vi "GetMUXRelayInfo.vi"(8 "error in (no error)":errorcluster, 10 "gRPCid":T2, 11 "ctet_mux in":T1) -> (0 "error out":errorcluster, 3 "ctet_mux out":T1)   [LabVIEW 2019, in "ctet_mux_User Library.lvlib"]
uses:
  ctet_mux_User Library.lvlib
  Servers/ctet_mux/gRPC lvSupport/Server API/typeDefs/grpcId.ctl
  Types/ctet_mux.ctl
  Servers/ctet_mux/ctet_mux Class/RPC Messages/measurementservice_MUXGetRelayInfoResponse/measurementservice_MUXGetRelayInfoResponse_Data.ctl
  Servers/ctet_mux/ctet_mux Class/RPC Messages/measurementservice_RelayInfoCluster/measurementservice_RelayInfoCluster_Data.ctl
  Servers/ctet_mux/ctet_mux Class/RPC Messages/measurementservice_ErrorOut/measurementservice_ErrorOut_Data.ctl
  Servers/ctet_mux/ctet_mux Class/ctet_mux.lvclass
  Servers/ctet_mux/gRPC lvSupport/gprc-lvsupport.lvlib
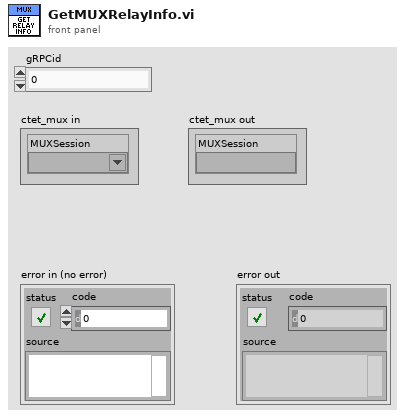
[diagram p1: front panel]
types:
  T1 = typedef "ctet_mux_User Library.lvlib/ctet_mux.ctl" = cluster{"MUXSession":refnum<k15>}
  T2 = typedef "ctet_mux.lvlib/gprc-lvsupport.lvlib/grpcId.ctl" = u64
  T3 = typedef "ctet_mux.lvlib/ctet_mux.lvclass/measurementservice_ErrorOut_Data.ctl" = cluster{"errCode":i64, "errMessage":string}
  T4 = typedef "ctet_mux.lvlib/ctet_mux.lvclass/measurementservice_MUXGetRelayInfoResponse_Data.ctl" = cluster{"RelayInfo":T5[], "error":T3}
  T5 = typedef "ctet_mux.lvlib/ctet_mux.lvclass/measurementservice_RelayInfoCluster_Data.ctl" = cluster{"RelayName":string, "RelayCount":i64}
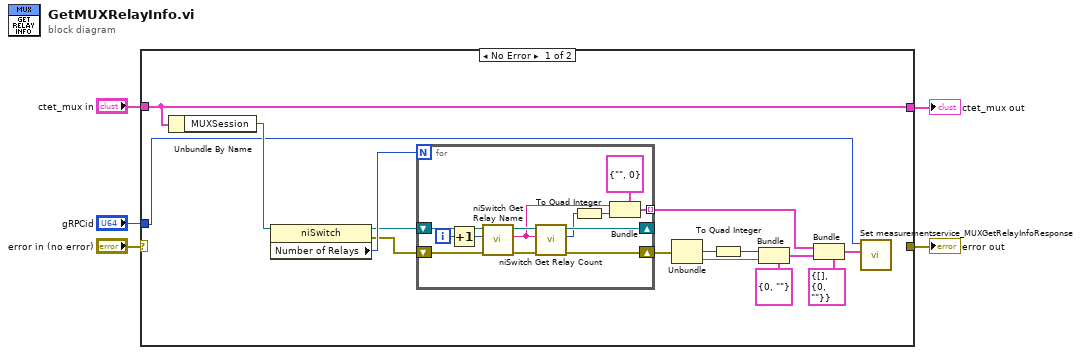
[diagram p0: block diagram]
diagram:
  n1 = case shown="No Error" "error in (no error)" {
    selector: "error in (no error)" -> [_ w35]
    tunnel: [_ w35] -> w5
    tunnel: "gRPCid" -> [w15 _]
    tunnel: "ctet_mux in" -> [w17 w34]
    tunnel: [w17 w34] -> w1
    frame No Error {
      n2 = Unbundle By Name(w17) -> ("MUXSession"=w16:refnum<k15>)
      n3 = property class="niSwitch"(reference=w16) -> (reference out=w9:refnum<k15>, error out=w8:errorcluster, "Number of Relays"=w10:i32)  [unwired: 1 in]
      n4 = for {
        N: w10 -> [_]
        shift-right: [w29] -> _
        shift-left: w9 -> [w33]
        shift-right: [w28] -> w7
        shift-left: w8 -> [w32]
        tunnel: [w21] -> w6 mode=indexing
        i -> [w27]
        n5 = Increment(x=w27) -> (x+1=w26:i32)
        n6 = call <instrlib>:"niSwitch Get Relay Name.vi"("error in (no error)"=w32, "index (1)"=w26, "instrument handle"=w33) -> ("error out"=w30:errorcluster, "relay name"=w24:string, "instrument handle out"=w31:refnum<k15>)  [unwired: 6 in]
        n7 = call <instrlib>:"niSwitch Get Relay Count.vi"("error in (no error)"=w30, "relay name"=w24, "instrument handle"=w31) -> ("error out"=w28:errorcluster, "count"=w23:i32, "instrument handle out"=w29:refnum<k15>)  [unwired: 6 in]
        n8 = To Quad Integer(1:w23) -> (0:w22:i64)
        n9 = Bundle(cluster=T5 {"RelayName"="", "RelayCount"=0} ("measurementservice_RelayInfoCluster_Data"), "RelayName"=w24, "RelayCount"=w22) -> (w21:T5)
      }
      n10 = Unbundle(w7) -> ("code"=w19:i32, "source"=w20:string)  [unwired: 1 out]
      n11 = To Quad Integer(1:w19) -> (0:w18:i64)
      n12 = Bundle(cluster=T3 {"errCode"=0, "errMessage"=""} ("error"), "errCode"=w18, "errMessage"=w20) -> (w11:T3)
      n13 = Bundle(cluster=T4 {"RelayInfo"=[], "error"={"errCode"=0, "errMessage"=""}} ("measurementservice_MUXGetRelayInfoResponse_Data"), "RelayInfo"=w6, "error"=w11) -> (w13:T4)
      n14 = call "Set measurementservice_MUXGetRelayInfoResponse.vi"("Message Data"=w13, "gRPCid"=w15) -> ()  [unwired: 9 in, 1 out]
    }
    frame Error {
    }
  }
  "error out" <- w5
  "ctet_mux out" <- w1
